vi "Data_PSD_287.vi"() -> ()   [LabVIEW 2020]
uses:
  <vilib>/Utility/error.llb/DialogType.ctl
  <vilib>/measure/maspectr.llb/Power Spectrum and PSD Export Mode.ctl
  <vilib>/Analysis/4window.llb/windowTd.ctl
  <vilib>/sound2/lvsound2.llb/Sound File Info (path).vi
  <vilib>/measure/maspectr.llb/FFT Power Spectrum and PSD for 1 Chan.vi
  <vilib>/Analysis/0measdsp.llb/Scaled Time Domain Window (DBL).vi
  <vilib>/sound2/lvsound2.llb/Sound File Read Open.vi
  <vilib>/sound2/lvsound2.llb/Sound File Read (DBL).vi
  <vilib>/Analysis/NI_AALPro.lvlib
  <vilib>/measure/NI_MAPro.lvlib
panel:
  in  "Stop Button":bool
  out "Data Cursor":T1
  in  "File Path":path
  out "Max Amplitude":dbl
  out "Frequency Peak":dbl
  out "Signal":waveform(dbl)(graph)
  out "PSD of Signal":cluster{"f0":dbl, "df":dbl, "magnitude":dbl[]}(graph)
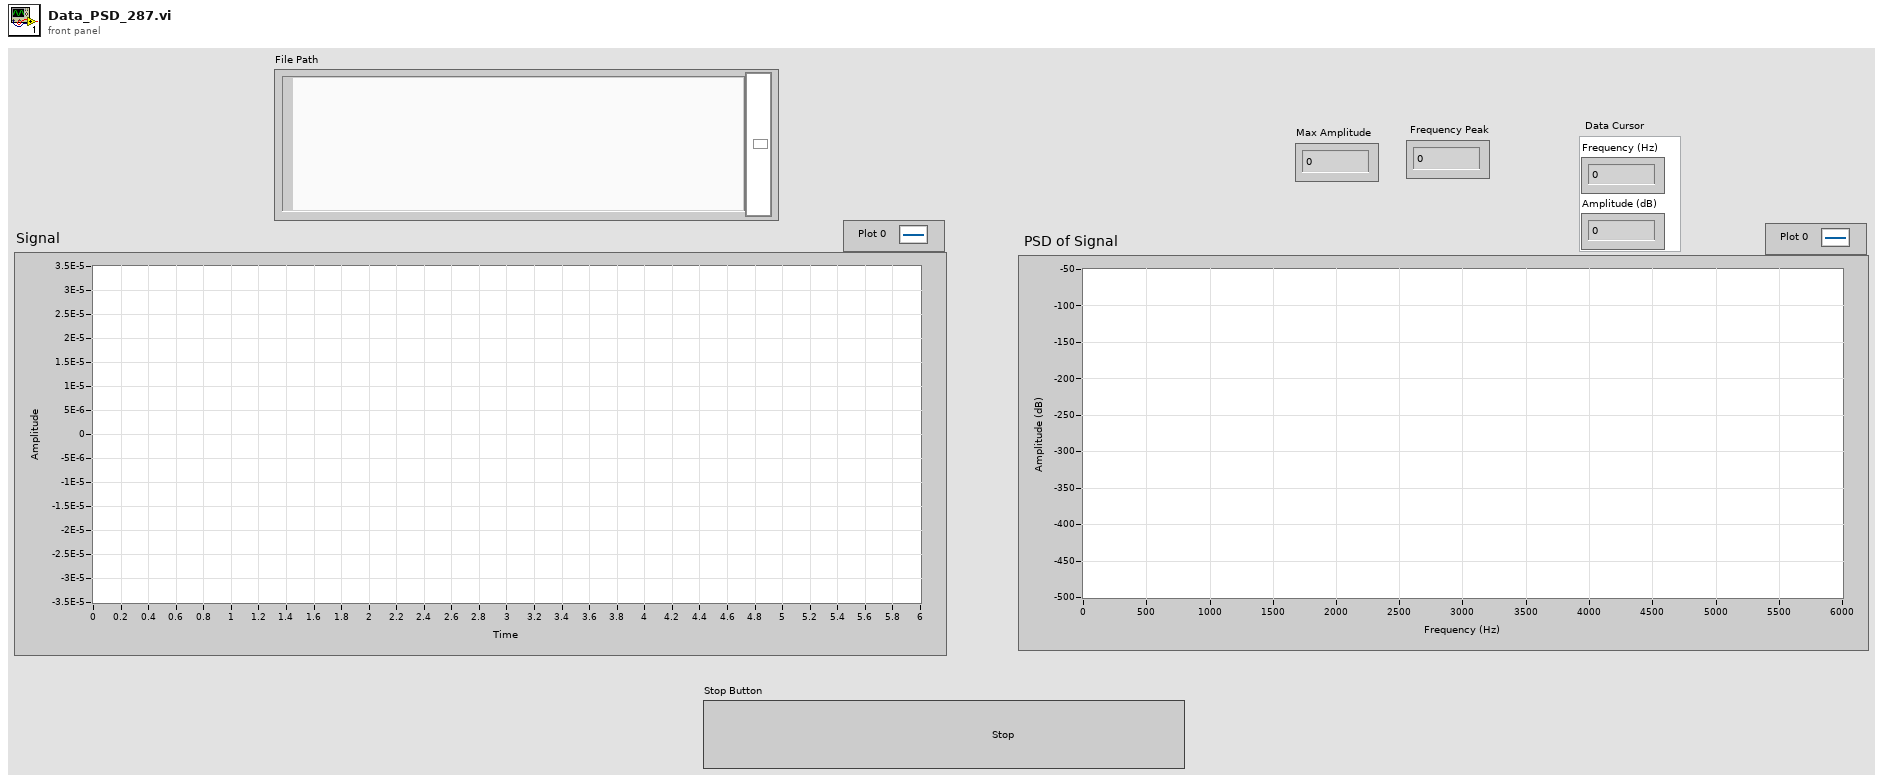
[diagram p1: front panel]
types:
  T1 = cluster{"Frequency (Hz)":dbl, "Amplitude (dB)":dbl}
  T2 = cluster{"Data":dbl[], "ctl":enum16{"Init", "Exit"}}
  T3 = typedef "DialogType.ctl" = u16
  T4 = typedef "NI_AALPro.lvlib/windowTd.ctl" = u32
  T5 = typedef "NI_MAPro.lvlib/Power Spectrum and PSD Export Mode.ctl" = u16
  T6 = typedef "Sound File Refnum.ctl" = refnum<file>
  T7 = typedef "LVPointDoubleTypeDef.ctl" = cluster{"Cursor X":dbl, "Cursor Y":dbl}
  T8 = typedef "LVRangeTypeDef.ctl" = cluster{"Minimum":dbl, "Maximum":dbl, "Increment":dbl, "Minor Increment":dbl, "Start":dbl}
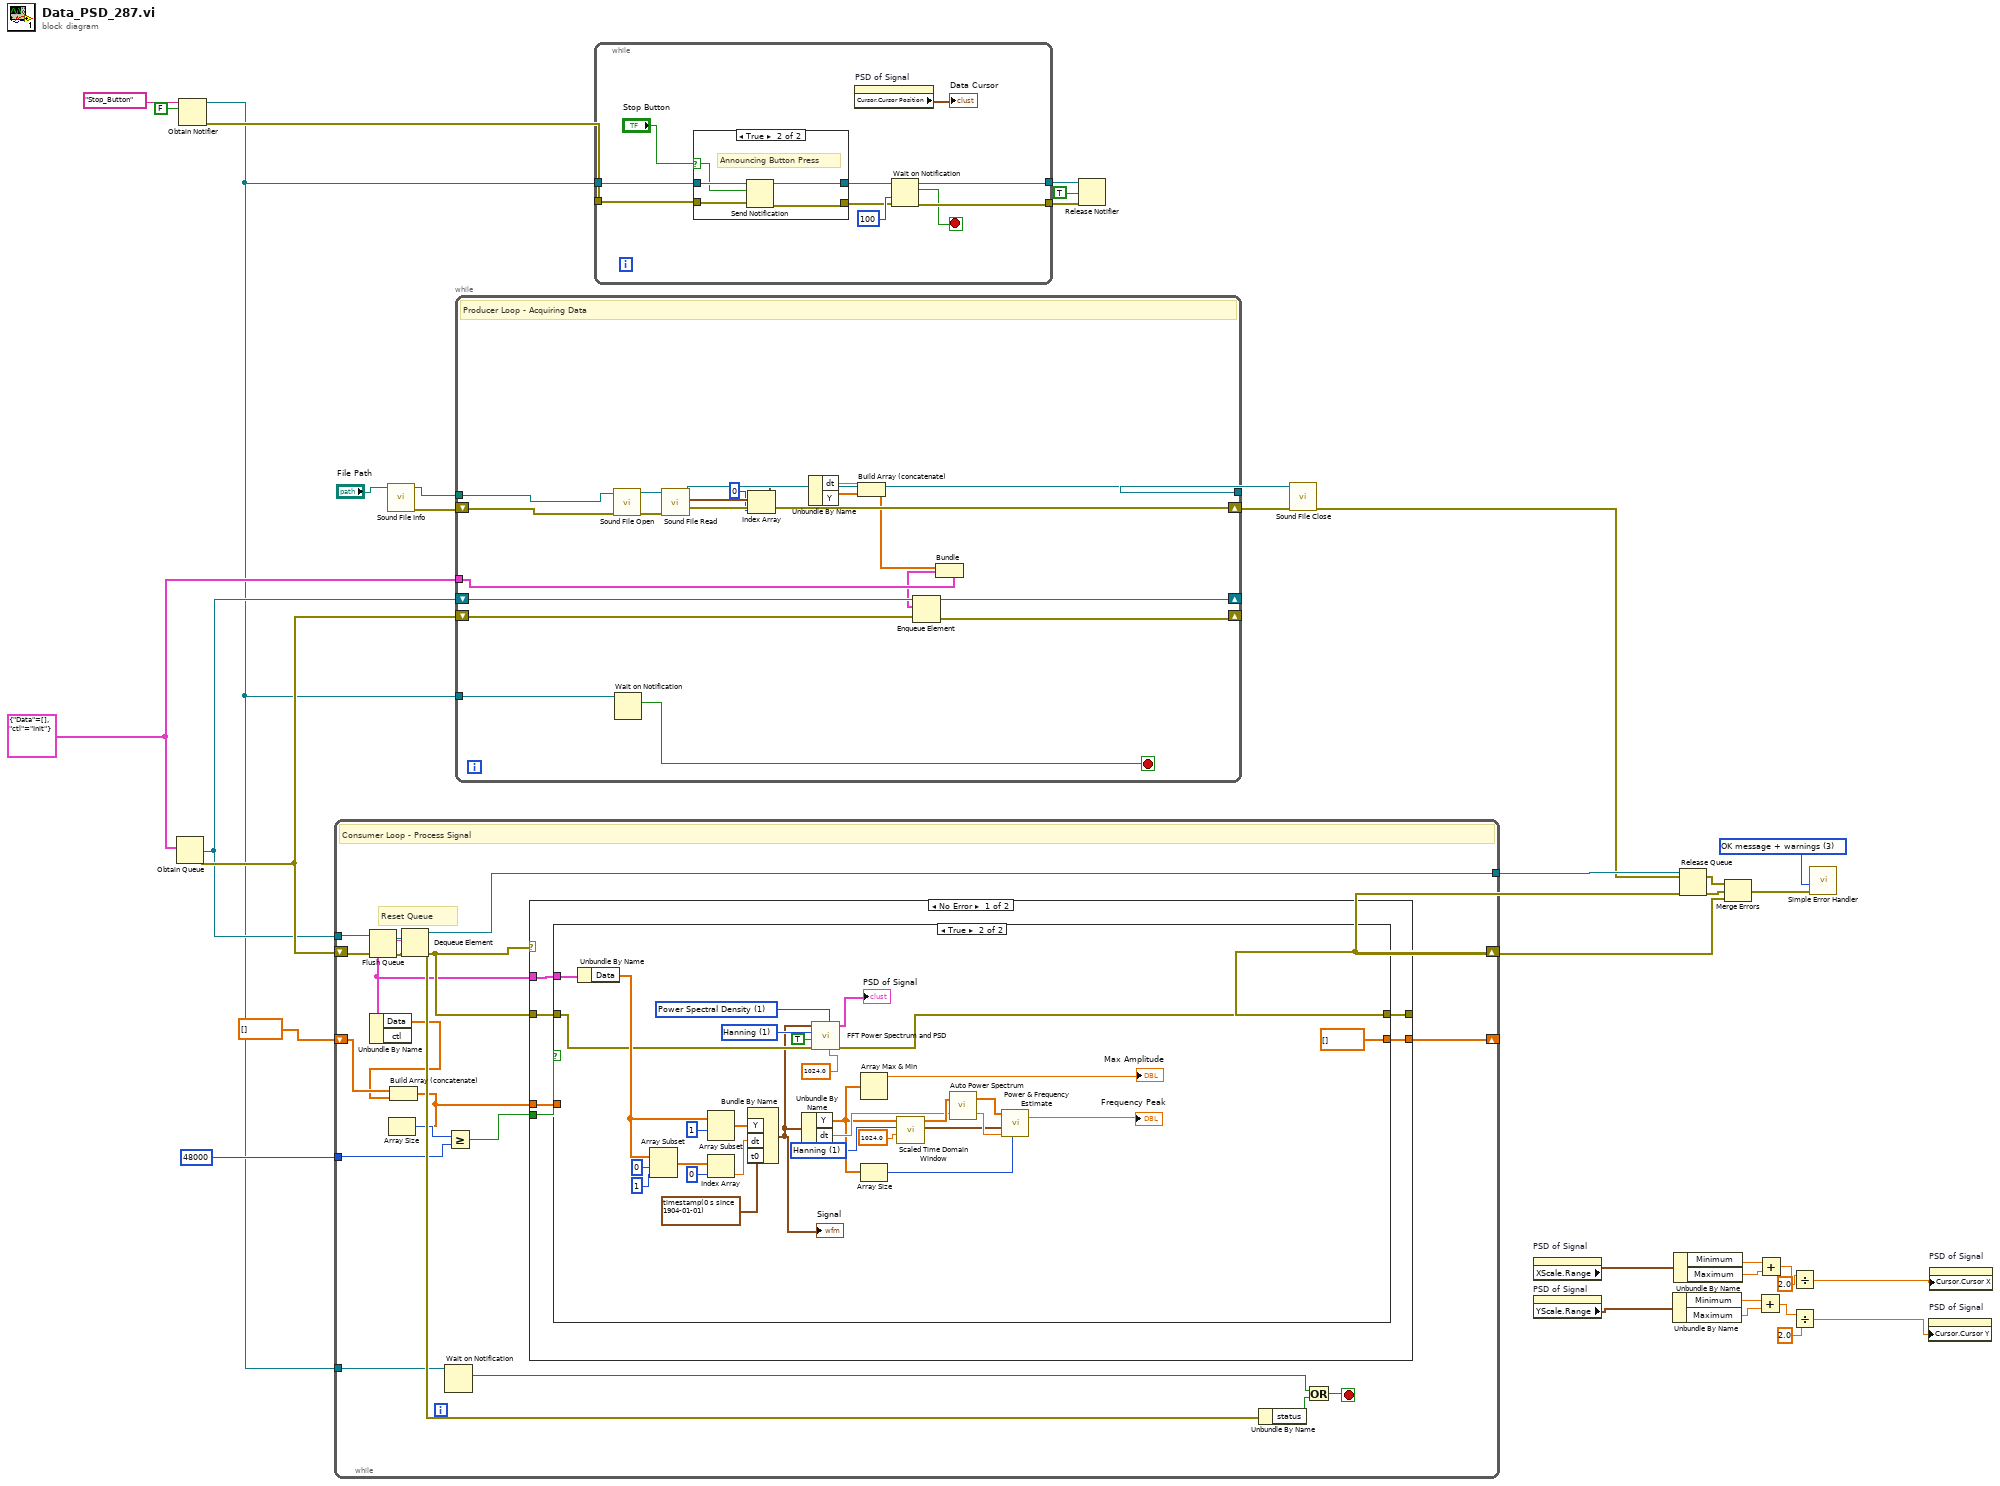
[diagram p0: block diagram]
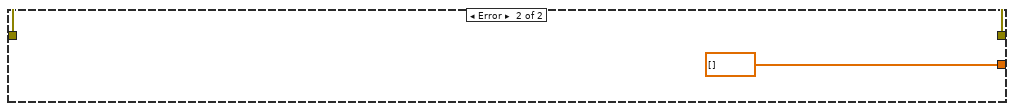
[diagram p4: hidden frame]
diagram:
  w20 = T2 {"Data"=[], "ctl"=enum."Init"}
  w35 = T3 3 items=["no dialog", "OK message", "continue or stop message", "OK message + warnings", "continue/stop + warnings"] ("type of dialog (OK msg:1)")
  n1 = Obtain Queue(element data type=w20) -> (queue out=w24:refnum<queue>, error out=w25:errorcluster)  [unwired: 3 in, 2 out]
  n2 = Obtain Notifier(name (unnamed)="Stop_Button", notification data type=FALSE) -> (notifier out=w14:refnum<notifier>, error out=w15:errorcluster)  [unwired: 2 in, 1 out]
  n3 = while {
    tunnel: w24 -> [w51]
    shift-right: [w54] -> w32
    shift-left: w25 -> [w49]
    tunnel: [w47] -> w33
    tunnel: 48000 -> [w43]
    shift-right: [w39] -> _
    shift-left: dbl[] [] -> [w44]
    tunnel: w14 -> [w37]
    stop <- w52 stop-if-true
    # "Reset Queue"
    # "Consumer Loop - Process Signal"
    n4 = Flush Queue(queue=w51, error in (no error)=w49) -> (queue out=w50:refnum<queue>, error out=w48:errorcluster)  [unwired: 1 out]
    n5 = Dequeue Element(queue=w50, error in (no error)=w48) -> (queue out=w47:refnum<queue>, element=w45:T2, error out=w46:errorcluster)  [unwired: 2 out]
    n6 = Unbundle By Name(w45) -> ("Data"=w40:dbl[])  [unwired: 1 out]
    n7 = Build Array (concatenate)(w44, w40) -> (w38:dbl[])
    n8 = Array Size(array=w38) -> (size(s)=w42:i32)
    n9 = Wait on Notification(notifier=w37) -> (notification=w36:bool)  [unwired: 3 in, 3 out]
    n10 = Greater Or Equal?(x=w42, y=w43) -> (x >= y?=w41:bool)
    n11 = case shown="No Error" w46 {
      tunnel: w45 -> [w60 _]
      tunnel: [w55 w94] -> w54
      tunnel: w46 -> [w56 w94]
      tunnel: w41 -> [w59 _]
      tunnel: [w58 dbl[] []] -> w39
      tunnel: w38 -> [w57 _]
      frame No Error {
        n12 = case shown="True" w59 {
          tunnel: w60 -> [_ w74]
          tunnel: [w62 dbl[] []] -> w58
          tunnel: w57 -> [w62 _]
          tunnel: w56 -> [w61 w70]
          tunnel: [w61 w69] -> w55
          frame False {
          }
          frame True {
            w75 = T4 1 items=["Rectangle"=0, "Hanning"=1, "Hamming"=2, "Blackman-Harris"=3, "Exact Blackman"=4, "Blackman"=5, "Flat Top"=6, "4 Term B-Harris "=7, "7 Term B-Harris"=8, "Low Sidelobe"=9, "Blackman Nuttall"=11, "Triangle"=30, "Bartlett-Hanning"=31, "Bohman"=32, "Parzen"=33, "Welch"=34, "Kaiser"=60, "Dolph-Chebyshev"=61, "Gaussian"=62] ("window")
            w76 = T4 1 items=["Rectangle"=0, "Hanning"=1, "Hamming"=2, "Blackman-Harris"=3, "Exact Blackman"=4, "Blackman"=5, "Flat Top"=6, "4 Term B-Harris "=7, "7 Term B-Harris"=8, "Low Sidelobe"=9, "Blackman Nuttall"=11, "Triangle"=30, "Bartlett-Hanning"=31, "Bohman"=32, "Parzen"=33, "Welch"=34, "Kaiser"=60, "Dolph-Chebyshev"=61, "Gaussian"=62] ("window")
            w89 = T5 1 items=["Power Spectrum", "Power Spectral Density"] ("export mode")
            n13 = Unbundle By Name(w74) -> ("Data"=w73:dbl[])
            n14 = Array Subset(array=w73, index=0, length=1) -> (w85:dbl[])
            n15 = Array Subset(array=w73, index=1) -> (w86:dbl[])  [unwired: 1 in]
            n16 = Index Array(array=w85, index=0) -> (element=w83:dbl)
            n17 = Bundle By Name("Y"=w86, "dt"=w83, "t0"=timestamp(0 s since 1904-01-01)) -> (w63:waveform(dbl))  [unwired: 1 in]
            "Signal" <- w63
            n18 = Unbundle By Name(w63) -> ("Y"=w79:dbl[], "dt"=w88:dbl)
            n19 = call-poly <vilib>:"FFT Power Spectrum and PSD.vi"("window parameter"=1024.0, "export mode"=w89, "error in (no error)"=w70, "dB On (F)"=TRUE, "window"=w75, "time signal"=w63) -> ("error out"=w69:errorcluster, "Power Spectrum / PSD"=→"PSD of Signal":cluster{"f0":dbl, "df":dbl, "magnitude":dbl[]})  [unwired: 2 in, 2 out]
            n20 = Array Max & Min(array=w79) -> (max value=→"Max Amplitude":dbl)  [unwired: 3 out]
            n21 = Array Size(array=w79) -> (size(s)=w78:i32)
            n22 = call-poly <vilib>:"Scaled Time Domain Window.vi"("window parameter"=1024.0, "window"=w76, "X"=w79) -> ("window properties"=w77:cluster{"eq noise BW":dbl, "coherent gain":dbl}, "Windowed X"=w91:dbl[])  [unwired: 7 out]
            n23 = call <vilib>:"Auto Power Spectrum.vi"("dt"=w88, "Signal (V)"=w91) -> ("df"=w92:dbl, "Power Spectrum (V^2 rms)"=w80:dbl[])
            n24 = call <vilib>:"Power & Frequency Estimate.vi"("span"=w78, "df"=w92, "window constants"=w77, "Power Spectrum (V^2 rms)"=w80) -> ("est frequency peak"=→"Frequency Peak":dbl)  [unwired: 1 in, 2 out]
          }
        }
      }
      frame Error {
      }
    }
    n25 = Unbundle By Name(w46) -> ("status"=w53:bool)
    n26 = Or(x=w36, y=w53) -> (x .or. y?=w52:bool)
  }
  n27 = call-poly <vilib>:"Sound File Info.vi"("path"="File Path") -> ("error out"=w28:errorcluster, "path out"=w29:path)  [unwired: 7 in, 2 out]
  n28 = while {
    shift-right: [w113] -> _
    shift-left: w25 -> [w114]
    shift-right: [w109] -> w26
    shift-left: w28 -> [w111]
    tunnel: w29 -> [w112]
    tunnel: [w110] -> w27
    shift-right: [w107] -> _
    shift-left: w24 -> [w108]
    tunnel: w20 -> [w106]
    tunnel: w14 -> [w96]
    stop <- w95 stop-if-true
    # "Producer Loop - Acquiring Data"
    n29 = call-poly <vilib>:"Sound File Open.vi"("error in (no error)"=w111, "path"=w112) -> ("error out"=w104:errorcluster, "sound file refnum"=w105:T6)  [unwired: 8 in]
    n30 = Wait on Notification(notifier=w96) -> (notification=w95:bool)  [unwired: 3 in, 3 out]
    n31 = call-poly <vilib>:"Sound File Read.vi"("error in (no error)"=w104, "sound file refnum"=w105) -> ("error out"=w109:errorcluster, "data"=w103:waveform(dbl)[], "sound file refnum out"=w110:T6)  [unwired: 5 in, 2 out]
    n32 = Index Array(array=w103, index=0) -> (element=w101:waveform(dbl))
    n33 = Unbundle By Name(w101) -> ("dt"=w100:dbl, "Y"=w99:dbl[])
    n34 = Build Array (concatenate)(w100, w99) -> (w98:dbl[])
    n35 = Bundle(cluster=w106, "Data"=w98) -> (w97:T2)  [unwired: 1 in]
    n36 = Enqueue Element(queue=w108, element=w97, error in (no error)=w114) -> (queue out=w107:refnum<queue>, error out=w113:errorcluster)  [unwired: 2 out]
  }
  n37 = while {
    tunnel: w15 -> [w124]
    tunnel: w14 -> [w122]
    tunnel: [w119] -> w16
    tunnel: [w118] -> w17
    stop <- w117 stop-if-true
    n38 = case shown="True" "Stop Button" {
      selector: "Stop Button" -> [_ w127]
      tunnel: w124 -> [w125 w131]
      tunnel: w122 -> [w126 w130]
      tunnel: [w126 w129] -> w121
      tunnel: [w125 w128] -> w120
      frame False {
      }
      frame True {
        # "Announcing Button Press"
        n39 = Send Notification(notification=w127, notifier=w130, error in (no error)=w131) -> (notifier out=w129:refnum<notifier>, error out=w128:errorcluster)
      }
    }
    n40 = property on="PSD of Signal" class="WFGraph (strict)"() -> ("Cursor.Cursor Position"=→"Data Cursor":T7)  [unwired: 2 in, 2 out]
    n41 = Wait on Notification(notifier=w121, timeout in ms (-1)=100, error in (no error)=w120) -> (notifier out=w118:refnum<notifier>, notification=w117:bool, error out=w119:errorcluster)  [unwired: 1 in, 1 out]
  }
  n42 = Release Notifier(notifier=w17, force destroy? (F)=TRUE, error in (no error)=w16) -> ()  [unwired: 3 out]
  n43 = call <vilib>:"Sound File Close.vi"("error in (no error)"=w26, "sound file refnum"=w27) -> ("error out"=w23:errorcluster)  [unwired: 9 in]
  n44 = property on="PSD of Signal" class="WFGraph (strict)"() -> ("XScale.Range"=w1:T8)  [unwired: 2 in, 2 out]
  n45 = property on="PSD of Signal" class="WFGraph (strict)"() -> ("YScale.Range"=w2:T8)  [unwired: 2 in, 2 out]
  n46 = Unbundle By Name(w2) -> ("Minimum"=w6:dbl, "Maximum"=w5:dbl)
  n47 = Unbundle By Name(w1) -> ("Minimum"=w12:dbl, "Maximum"=w11:dbl)
  n48 = Release Queue(queue=w33, error in (no error)=w32) -> (error out=w31:errorcluster)  [unwired: 1 in, 2 out]
  n49 = Merge Errors(w23, w31, w32) -> (w34:errorcluster)
  n50 = Add(x=w6, y=w5) -> (x+y=w8:dbl)
  n51 = Add(x=w12, y=w11) -> (x+y=w9:dbl)
  n52 = Divide(x=2.0 ("y"), y=w9) -> (x/y=w3:dbl)
  n53 = Divide(x=w8, y=2.0) -> (x/y=w4:dbl)
  n54 = call <vilib>:"Simple Error Handler.vi"("type of dialog (OK msg:1)"=w35, "error in (no error)"=w34) -> ()  [unwired: 8 out]
  n55 = property on="PSD of Signal" class="WFGraph (strict)"("Cursor.Cursor Y"=w4) -> ()  [unwired: 2 in, 2 out]
  n56 = property on="PSD of Signal" class="WFGraph (strict)"("Cursor.Cursor X"=w3) -> ()  [unwired: 2 in, 2 out]
